vi "plot matrix averages.vi"(11 "2D array":dbl[][](array[numeric])) -> (3 "transposed array":dbl[][](array[numeric]))   [LabVIEW 2013]
uses:
  <vilib>/gmath/statdist.llb/st_Percentiles (scalar).vi
  <vilib>/Analysis/NI_AALBase.lvlib
  <vilib>/gmath/NI_Gmath.lvlib
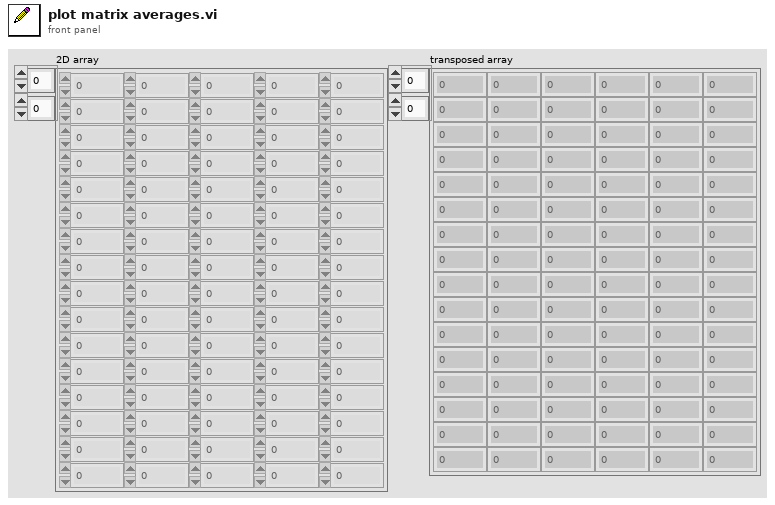
[diagram p1: front panel]
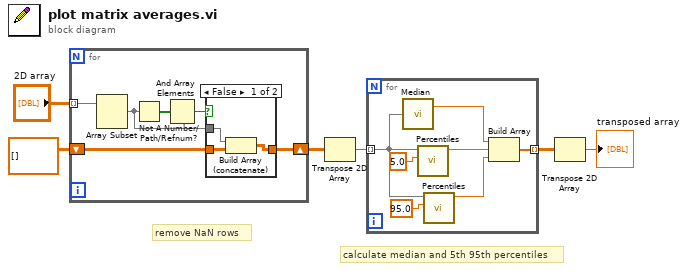
[diagram p0: block diagram]
diagram:
  # "calculate median and 5th 95th percentiles"
  # "remove NaN rows"
  n1 = for {
    tunnel: "2D array" -> [w12] mode=indexing
    shift-right: [w8] -> w1
    shift-left: dbl[][] [] -> [w7]
    n2 = Array Subset(array=w12) -> (w9:dbl[])  [unwired: 2 in]
    n3 = Not A Number/Path/Refnum?(number/path/refnum=w9) -> (NaN/Path/Refnum?=w11:bool[])
    n4 = And Array Elements(Boolean array=w11) -> (logical AND=w10:bool)
    n5 = case shown="False" w10 {
      tunnel: w7 -> [w15 w16]
      tunnel: w9 -> [w14 _]
      tunnel: [w13 w16] -> w8
      frame False {
        n6 = Build Array (concatenate)(w14, w15) -> (w13:dbl[][])
      }
      frame True {
      }
    }
  }
  n7 = Transpose 2D Array(2D array=w1) -> (transposed array=w5:dbl[][])
  n8 = for {
    tunnel: w5 -> [w23] mode=indexing
    tunnel: [w17] -> w6 mode=indexing
    n9 = call <vilib>:"Median.vi"("X"=w23) -> ("median"=w22:dbl)  [unwired: 1 out]
    n10 = call-poly <vilib>:"Percentiles.vi"("p"=5.0, "x array"=w23) -> ("percentile"=w21:dbl)  [unwired: 8 in, 1 out]
    n11 = call-poly <vilib>:"Percentiles.vi"("p"=95.0, "x array"=w23) -> ("percentile"=w20:dbl)  [unwired: 8 in, 1 out]
    n12 = Build Array(w22, w21, w20) -> (w17:dbl[])
  }
  n13 = Transpose 2D Array(2D array=w6) -> (transposed array=→"transposed array":dbl[][])
